vi "read_log.vi"() -> ()   [LabVIEW 2013]
panel:
  in  "milliseconds to wait":u32
  out "record(s)":T1(array[cluster])
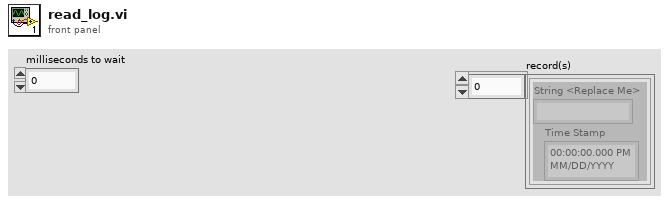
[diagram p1: front panel]
types:
  T1 = cluster{"String <Replace Me>":string, "Time Stamp":timestamp}[]
  T2 = cluster{"String <Replace Me>":string, "Time Stamp":timestamp}
  T3 = enum16{"open", "replace", "create", "open or create", "replace or create", "replace or create with confirmation"}
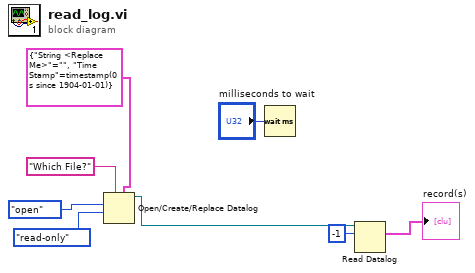
[diagram p0: block diagram]
diagram:
  n1 = Open/Create/Replace Datalog(5:T2 {"String <Replace Me>"="", "Time Stamp"=timestamp(0 s since 1904-01-01)} ("Data"), 7:"Which File?" ("prompt"), 9:enum16{"read/write", "read-only", "write-only"}."read-only" ("access (0:read/write)"), 10:T3."open" ("operation (0:open)")) -> (3:w4:refnum<k1>)  [unwired: 2 in, 2 out]
  n2 = Wait (ms)(milliseconds to wait="milliseconds to wait") -> ()  [unwired: 1 out]
  n3 = Read Datalog(6:-1 ("count (1)"), 7:w4) -> (2:→"record(s)":T1)  [unwired: 1 in, 2 out]
